vi "uStringManipulation_addPrefix_Set.vi"(8 "error in (no error)":errorcluster, 10 "prefix":string, 11 "addPrefix in":refnum<class "addPrefix.lvclass">) -> (0 "error out":errorcluster, 3 "addPrefix out":refnum<class "addPrefix.lvclass">)   [LabVIEW 2021, in "uStringManipulation_Pack_Std.lvlib" / "addPrefix.lvclass"]
doc: "Set a prefix to prepend at the beginning of the string."
uses:
  addPrefix.lvclass
  addPrefix.lvclass/addPrefix.ctl
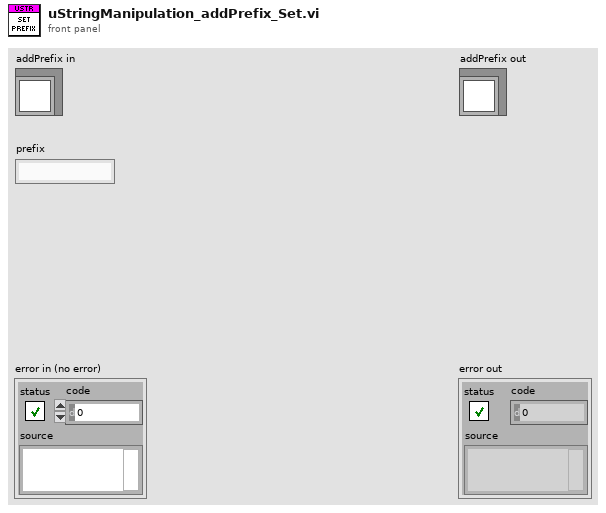
[diagram p1: front panel]
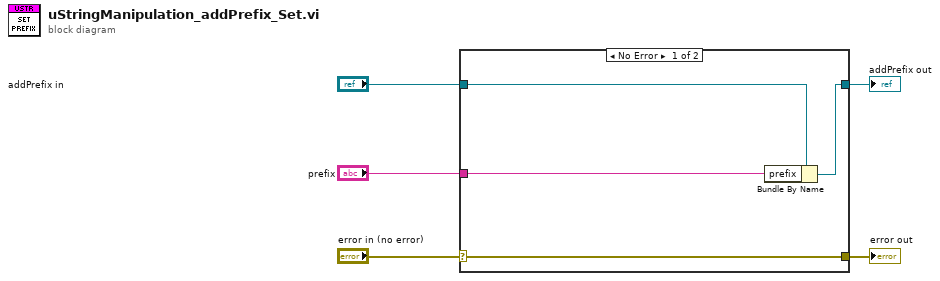
[diagram p0: block diagram]
diagram:
  n1 = case shown="No Error" "error in (no error)" {
    selector: "error in (no error)" -> [w9 w10]
    tunnel: [w9 w10] -> w4
    tunnel: [w7 w11] -> w2
    tunnel: "addPrefix in" -> [w8 w11]
    tunnel: "prefix" -> [w6 _]
    frame No Error {
      n2 = Bundle By Name(cluster=w8, "prefix"=w6) -> (w7:refnum<class "addPrefix.lvclass">)
    }
    frame Error {
    }
  }
  "error out" <- w4
  "addPrefix out" <- w2
